vi "Get Node Attribute Map.vi"(11 "Refnum in":refnum<k20>) -> (3 "Map":map{string, string}(c390))   [LabVIEW 2021]
uses:
  <resource>/objmgr/DOMUserDefRef.rc
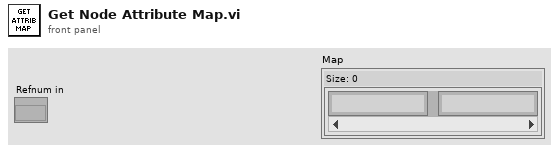
[diagram p1: front panel]
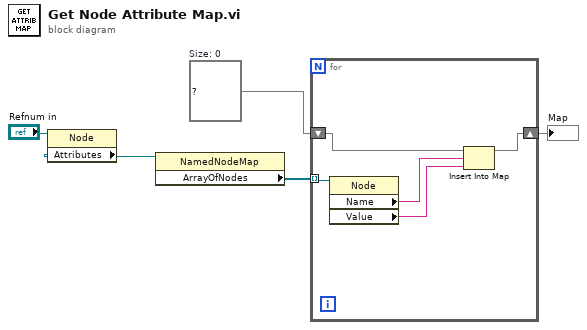
[diagram p0: block diagram]
diagram:
  w2 = map{string, string} {}  # Size: 0
  n1 = property class="Node"(reference="Refnum in") -> ("Attributes"=w4:refnum<k20>)  [unwired: 1 in, 2 out]
  n2 = property class="NamedNodeMap"(reference=w4) -> ("ArrayOfNodes"=w5:refnum<k20>[])  [unwired: 1 in, 2 out]
  n3 = for {
    tunnel: w5 -> [w10] mode=indexing
    shift-right: [w8] -> w1
    shift-left: w2 -> [w9]
    n4 = property class="Node"(reference=w10) -> ("Name"=w7:string, "Value"=w6:string)  [unwired: 1 in, 2 out]
    n5 = Insert Into Map(map in=w9, key=w7, value=w6) -> (map out=w8:map{string, string})  [unwired: 2 out]
  }
  "Map" <- w1
